vi "Read_Component_Power.vi"(8 "error in (no error)":errorcluster, 11 "AccelNET.lvlib:TCP.lvclass":refnum<class "TCP.lvclass">) -> (0 "Error Out":errorcluster, 2 "Component Power":T1)   [LabVIEW 2012, in "AccelNET.lvlib" / "TCP.lvclass"]
uses:
  TCP.lvclass
  Component_Power_Indicator.ctl
  Read_Selector.ctl
  Useful_Controls.lvlib
  Useful_SubVIs.lvlib
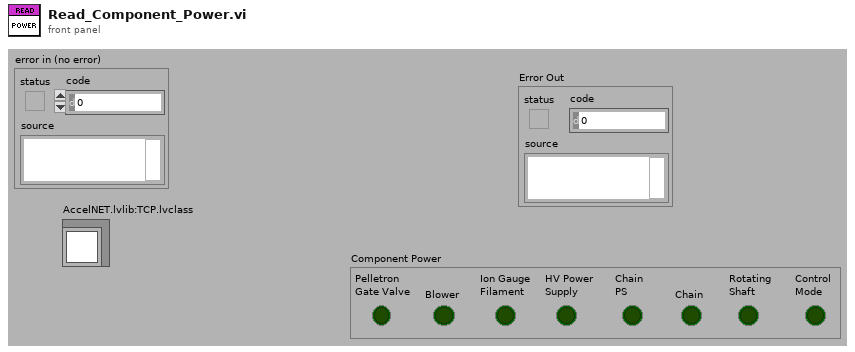
[diagram p1: front panel]
types:
  T1 = typedef "AccelNET.lvlib/Useful_Controls.lvlib/Component_Power_Indicator.ctl" = cluster{"Pelletron\nGate Valve":bool, "Blower":bool, "Chain":bool, "Rotating\nShaft":bool, "HV Power\nSupply":bool, "Ion Gauge\nFilament":bool, "Control\nMode":bool, "Chain\nPS":bool}
  T2 = typedef "AccelNET.lvlib/Useful_Controls.lvlib/Read_Selector.ctl" = u16
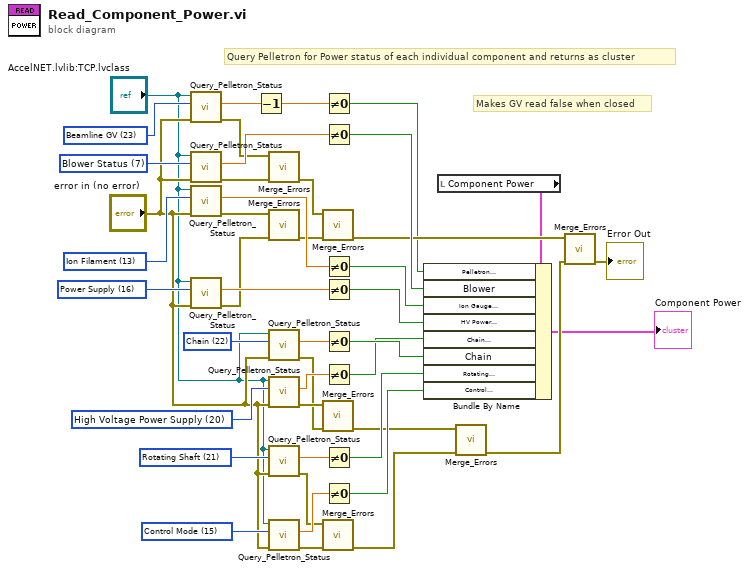
[diagram p0: block diagram]
diagram:
  w29 = T2 15 items=["Facility Key", "Chain Bypass", "Rotating Shaft Bypass", "Facility Interlock", "Pressure Interlock", "Temperature Interlock", "Water Flow Interlock", "Blower Status", "High Voltage", "+ High Voltage PS Readout", "- High Voltage PS Readout", "High Voltage PS Setting", "Ion Gauge", "Ion Filament", "Control Reference Voltage", "Control Mode", "Power Supply", "Chain Current", "Column Current", "Lost Current", "High Voltage Power Supply", "Rotating Shaft", "Chain", "Beamline GV", "Radiation", "Spark Count", "Spark Limit", "Spark Interlock"] ("Read Selector")
  w31 = T2 21 items=["Facility Key", "Chain Bypass", "Rotating Shaft Bypass", "Facility Interlock", "Pressure Interlock", "Temperature Interlock", "Water Flow Interlock", "Blower Status", "High Voltage", "+ High Voltage PS Readout", "- High Voltage PS Readout", "High Voltage PS Setting", "Ion Gauge", "Ion Filament", "Control Reference Voltage", "Control Mode", "Power Supply", "Chain Current", "Column Current", "Lost Current", "High Voltage Power Supply", "Rotating Shaft", "Chain", "Beamline GV", "Radiation", "Spark Count", "Spark Limit", "Spark Interlock"] ("Read Selector")
  w33 = T2 22 items=["Facility Key", "Chain Bypass", "Rotating Shaft Bypass", "Facility Interlock", "Pressure Interlock", "Temperature Interlock", "Water Flow Interlock", "Blower Status", "High Voltage", "+ High Voltage PS Readout", "- High Voltage PS Readout", "High Voltage PS Setting", "Ion Gauge", "Ion Filament", "Control Reference Voltage", "Control Mode", "Power Supply", "Chain Current", "Column Current", "Lost Current", "High Voltage Power Supply", "Rotating Shaft", "Chain", "Beamline GV", "Radiation", "Spark Count", "Spark Limit", "Spark Interlock"] ("Read Selector")
  w35 = T2 20 items=["Facility Key", "Chain Bypass", "Rotating Shaft Bypass", "Facility Interlock", "Pressure Interlock", "Temperature Interlock", "Water Flow Interlock", "Blower Status", "High Voltage", "+ High Voltage PS Readout", "- High Voltage PS Readout", "High Voltage PS Setting", "Ion Gauge", "Ion Filament", "Control Reference Voltage", "Control Mode", "Power Supply", "Chain Current", "Column Current", "Lost Current", "High Voltage Power Supply", "Rotating Shaft", "Chain", "Beamline GV", "Radiation", "Spark Count", "Spark Limit", "Spark Interlock"] ("Read Selector")
  w37 = T2 16 items=["Facility Key", "Chain Bypass", "Rotating Shaft Bypass", "Facility Interlock", "Pressure Interlock", "Temperature Interlock", "Water Flow Interlock", "Blower Status", "High Voltage", "+ High Voltage PS Readout", "- High Voltage PS Readout", "High Voltage PS Setting", "Ion Gauge", "Ion Filament", "Control Reference Voltage", "Control Mode", "Power Supply", "Chain Current", "Column Current", "Lost Current", "High Voltage Power Supply", "Rotating Shaft", "Chain", "Beamline GV", "Radiation", "Spark Count", "Spark Limit", "Spark Interlock"] ("Read Selector")
  w39 = T2 13 items=["Facility Key", "Chain Bypass", "Rotating Shaft Bypass", "Facility Interlock", "Pressure Interlock", "Temperature Interlock", "Water Flow Interlock", "Blower Status", "High Voltage", "+ High Voltage PS Readout", "- High Voltage PS Readout", "High Voltage PS Setting", "Ion Gauge", "Ion Filament", "Control Reference Voltage", "Control Mode", "Power Supply", "Chain Current", "Column Current", "Lost Current", "High Voltage Power Supply", "Rotating Shaft", "Chain", "Beamline GV", "Radiation", "Spark Count", "Spark Limit", "Spark Interlock"] ("Read Selector")
  w41 = T2 7 items=["Facility Key", "Chain Bypass", "Rotating Shaft Bypass", "Facility Interlock", "Pressure Interlock", "Temperature Interlock", "Water Flow Interlock", "Blower Status", "High Voltage", "+ High Voltage PS Readout", "- High Voltage PS Readout", "High Voltage PS Setting", "Ion Gauge", "Ion Filament", "Control Reference Voltage", "Control Mode", "Power Supply", "Chain Current", "Column Current", "Lost Current", "High Voltage Power Supply", "Rotating Shaft", "Chain", "Beamline GV", "Radiation", "Spark Count", "Spark Limit", "Spark Interlock"] ("Read Selector")
  w43 = T2 23 items=["Facility Key", "Chain Bypass", "Rotating Shaft Bypass", "Facility Interlock", "Pressure Interlock", "Temperature Interlock", "Water Flow Interlock", "Blower Status", "High Voltage", "+ High Voltage PS Readout", "- High Voltage PS Readout", "High Voltage PS Setting", "Ion Gauge", "Ion Filament", "Control Reference Voltage", "Control Mode", "Power Supply", "Chain Current", "Column Current", "Lost Current", "High Voltage Power Supply", "Rotating Shaft", "Chain", "Beamline GV", "Radiation", "Spark Count", "Spark Limit", "Spark Interlock"] ("Read Selector")
  # "Makes GV read false when closed"
  # "Query Pelletron for Power status of each individual component and returns as cluster"
  n1 = call "Query_Pelletron_Status.vi"("error in (no error)"="error in (no error)", "Read Selector"=w43, "AccelNET.lvlib:TCP.lvclass"="AccelNET.lvlib:TCP.lvclass") -> ("error out"=w20:errorcluster, "Data Out"=w44:dbl)  [unwired: 7 in]
  n2 = call "Query_Pelletron_Status.vi"("error in (no error)"="error in (no error)", "Read Selector"=w41, "AccelNET.lvlib:TCP.lvclass"="AccelNET.lvlib:TCP.lvclass") -> ("error out"=w19:errorcluster, "Data Out"=w42:dbl)  [unwired: 7 in]
  n3 = call "Query_Pelletron_Status.vi"("error in (no error)"="error in (no error)", "Read Selector"=w39, "AccelNET.lvlib:TCP.lvclass"="AccelNET.lvlib:TCP.lvclass") -> ("error out"=w18:errorcluster, "Data Out"=w40:dbl)  [unwired: 7 in]
  n4 = call "Query_Pelletron_Status.vi"("error in (no error)"="error in (no error)", "Read Selector"=w37, "AccelNET.lvlib:TCP.lvclass"="AccelNET.lvlib:TCP.lvclass") -> ("error out"=w17:errorcluster, "Data Out"=w38:dbl)  [unwired: 7 in]
  n5 = Decrement(x=w44) -> (x-1=w2:dbl)
  n6 = call "Merge_Errors.vi"("Error 2"=w19, "Error 1"=w20) -> ("Error Out"=w9:errorcluster)  [unwired: 9 in]
  n7 = call "Merge_Errors.vi"("Error 2"=w17, "Error 1"=w18) -> ("Error Out"=w10:errorcluster)  [unwired: 9 in]
  n8 = call "Query_Pelletron_Status.vi"("error in (no error)"="error in (no error)", "Read Selector"=w33, "AccelNET.lvlib:TCP.lvclass"="AccelNET.lvlib:TCP.lvclass") -> ("error out"=w15:errorcluster, "Data Out"=w34:dbl)  [unwired: 7 in]
  n9 = call "Query_Pelletron_Status.vi"("error in (no error)"="error in (no error)", "Read Selector"=w35, "AccelNET.lvlib:TCP.lvclass"="AccelNET.lvlib:TCP.lvclass") -> ("error out"=w16:errorcluster, "Data Out"=w36:dbl)  [unwired: 7 in]
  n10 = call "Query_Pelletron_Status.vi"("error in (no error)"="error in (no error)", "Read Selector"=w31, "AccelNET.lvlib:TCP.lvclass"="AccelNET.lvlib:TCP.lvclass") -> ("error out"=w14:errorcluster, "Data Out"=w32:dbl)  [unwired: 7 in]
  n11 = call "Query_Pelletron_Status.vi"("error in (no error)"="error in (no error)", "Read Selector"=w29, "AccelNET.lvlib:TCP.lvclass"="AccelNET.lvlib:TCP.lvclass") -> ("error out"=w13:errorcluster, "Data Out"=w30:dbl)  [unwired: 7 in]
  n12 = call "Merge_Errors.vi"("Error 2"=w10, "Error 1"=w9) -> ("Error Out"=w8:errorcluster)  [unwired: 9 in]
  n13 = call "Merge_Errors.vi"("Error 2"=w15, "Error 1"=w16) -> ("Error Out"=w12:errorcluster)  [unwired: 9 in]
  n14 = call "Merge_Errors.vi"("Error 2"=w13, "Error 1"=w14) -> ("Error Out"=w11:errorcluster)  [unwired: 9 in]
  n15 = Not Equal To 0?(x=w2) -> (x != 0?=w1:bool)
  n16 = Not Equal To 0?(x=w42) -> (x != 0?=w21:bool)
  n17 = Not Equal To 0?(x=w40) -> (x != 0?=w22:bool)
  n18 = Not Equal To 0?(x=w38) -> (x != 0?=w23:bool)
  n19 = Not Equal To 0?(x=w34) -> (x != 0?=w25:bool)
  n20 = Not Equal To 0?(x=w36) -> (x != 0?=w24:bool)
  n21 = Not Equal To 0?(x=w32) -> (x != 0?=w26:bool)
  n22 = Not Equal To 0?(x=w30) -> (x != 0?=w27:bool)
  n23 = local read "Component Power"() -> (w3:T1)
  n24 = Bundle By Name(cluster=w3, "Pelletron\nGate Valve"=w1, "Blower"=w21, "Ion Gauge\nFilament"=w22, "HV Power\nSupply"=w23, "Chain\nPS"=w24, "Chain"=w25, "Rotating\nShaft"=w26, "Control\nMode"=w27) -> (→"Component Power":T1)
  n25 = call "Merge_Errors.vi"("Error 2"=w11, "Error 1"=w12) -> ("Error Out"=w7:errorcluster)  [unwired: 9 in]
  n26 = call "Merge_Errors.vi"("Error 2"=w7, "Error 1"=w8) -> ("Error Out"=→"Error Out":errorcluster)  [unwired: 9 in]
